vi "decode_data.vi"(7 "offset":i32 min=0, 8 "error in (no error)":errorcluster, 9 "length":i32 min=0, 10 "encoded data string in":string, 11 "DL090602SutterMP285Stage in":refnum<class "StageDL090602SutterMP285.lvclass">) -> (0 "error out":errorcluster, 1 "decoded data":i32, 2 "encoded data string out":string, 3 "DL090602SutterMP285Stage out":refnum<class "StageDL090602SutterMP285.lvclass">)   [LabVIEW 2010, in "StageDL090602SutterMP285.lvclass"]
uses:
  StageDL090602SutterMP285.lvclass
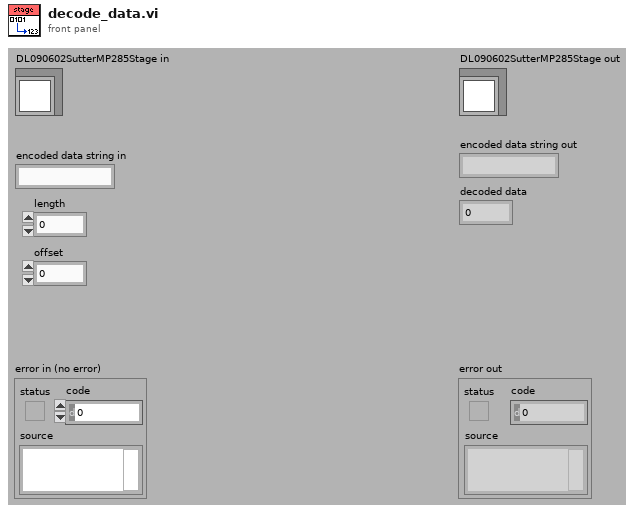
[diagram p1: front panel]
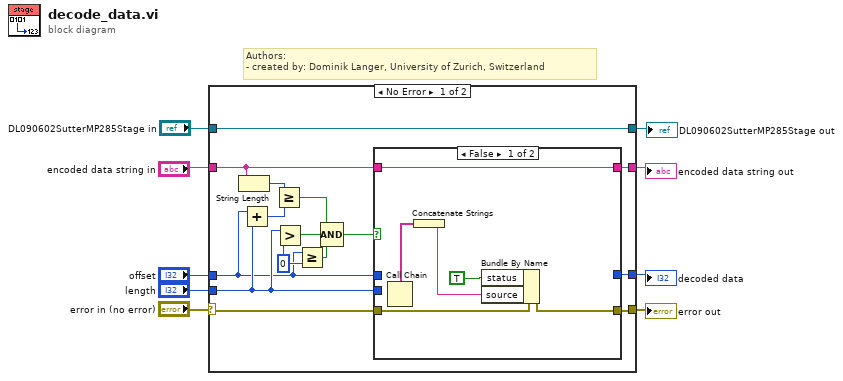
[diagram p0: block diagram]
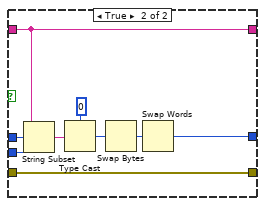
[diagram p2: hidden frame]
diagram:
  # "Authors: \n- created by: Dominik Langer, University of Zurich, Switzerland"
  n1 = case shown="No Error" "error in (no error)" {
    selector: "error in (no error)" -> [w17 w42]
    tunnel: [w16 w42] -> w8
    tunnel: [w24 w41] -> w6
    tunnel: "DL090602SutterMP285Stage in" -> [w24 w41]
    tunnel: [w15 w40] -> w5
    tunnel: "encoded data string in" -> [w10 w40]
    tunnel: [w14 _] -> w3
    tunnel: "offset" -> [w12 _]
    tunnel: "length" -> [w13 _]
    frame No Error {
      w20 = 0 ("offset")
      n2 = String Length(string=w10) -> (length=w18:i32)
      n3 = Add(x=w12, y=w13) -> (x+y=w19:i32)
      n4 = Greater Or Equal?(x=w18, y=w19) -> (x >= y?=w23:bool)
      n5 = Greater?(x=w13, y=w20) -> (0:w22:bool)
      n6 = Greater Or Equal?(x=w12, y=w20) -> (x >= y?=w21:bool)
      n7 = Compound Arithmetic op=AND(w23, w22, w21) -> (w11:bool)
      n8 = case shown="False" w11 {
        tunnel: w17 -> [w29 w35]
        tunnel: [w28 w35] -> w16
        tunnel: w10 -> [w30 w31]
        tunnel: w12 -> [_ w34]
        tunnel: w13 -> [_ w33]
        tunnel: [_ w32] -> w14
        tunnel: [w30 w31] -> w15
        frame False {
          n9 = Call Chain() -> (call chain=w26:string[])
          n10 = Concatenate Strings(w26) -> (w25:string)
          n11 = Bundle By Name(cluster=w29, "status"=TRUE, "source"=w25) -> (w28:errorcluster)
        }
        frame True {
          n12 = String Subset(string=w31, offset (0)=w34, length (rest)=w33) -> (substring=w37:string)
          n13 = Type Cast(type=0, x=w37) -> (*(type *) &x=w38:i32)
          n14 = Swap Bytes(anything=w38) -> (byte swapped=w39:i32)
          n15 = Swap Words(1:w39) -> (0:w32:i32)
        }
      }
    }
    frame Error {
    }
  }
  "error out" <- w8
  "DL090602SutterMP285Stage out" <- w6
  "encoded data string out" <- w5
  "decoded data" <- w3
